vi "main_ai.vi"() -> ()   [LabVIEW 2023]
uses:
  <vilib>/sound2/lvsound2.llb/Sound Output Set Volume (Single).vi
panel:
  in  "Reset":bool
  out "p2 score":i32
  out "p1 score":i32
  in  "Ball Speed":dbl(slide)=2.0 scale=0.0..5.0
  in  "Player Length":i32(slide)=100 scale=50.0..150.0
  in  "Pause Game":bool
  in  "Stop":bool
  in  "w_bool":bool
  in  "Down_bool":bool
  in  "s_bool":bool
  in  "Up_bool":bool
  out "game window":picture
  # "Player 1: W, S\nPlayer 2: Up, Down"
  # "Modifiers"
  # "Spacebar"
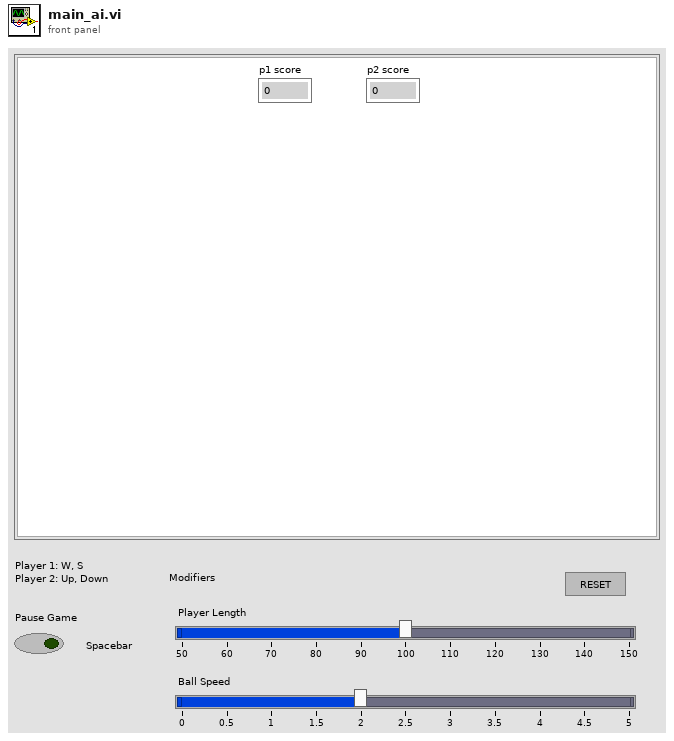
[diagram p1: front panel]
types:
  T1 = typedef "Sound Output Task ID.ctl" = u32
  T2 = cluster{"output vector x":dbl, "output vector y":dbl}
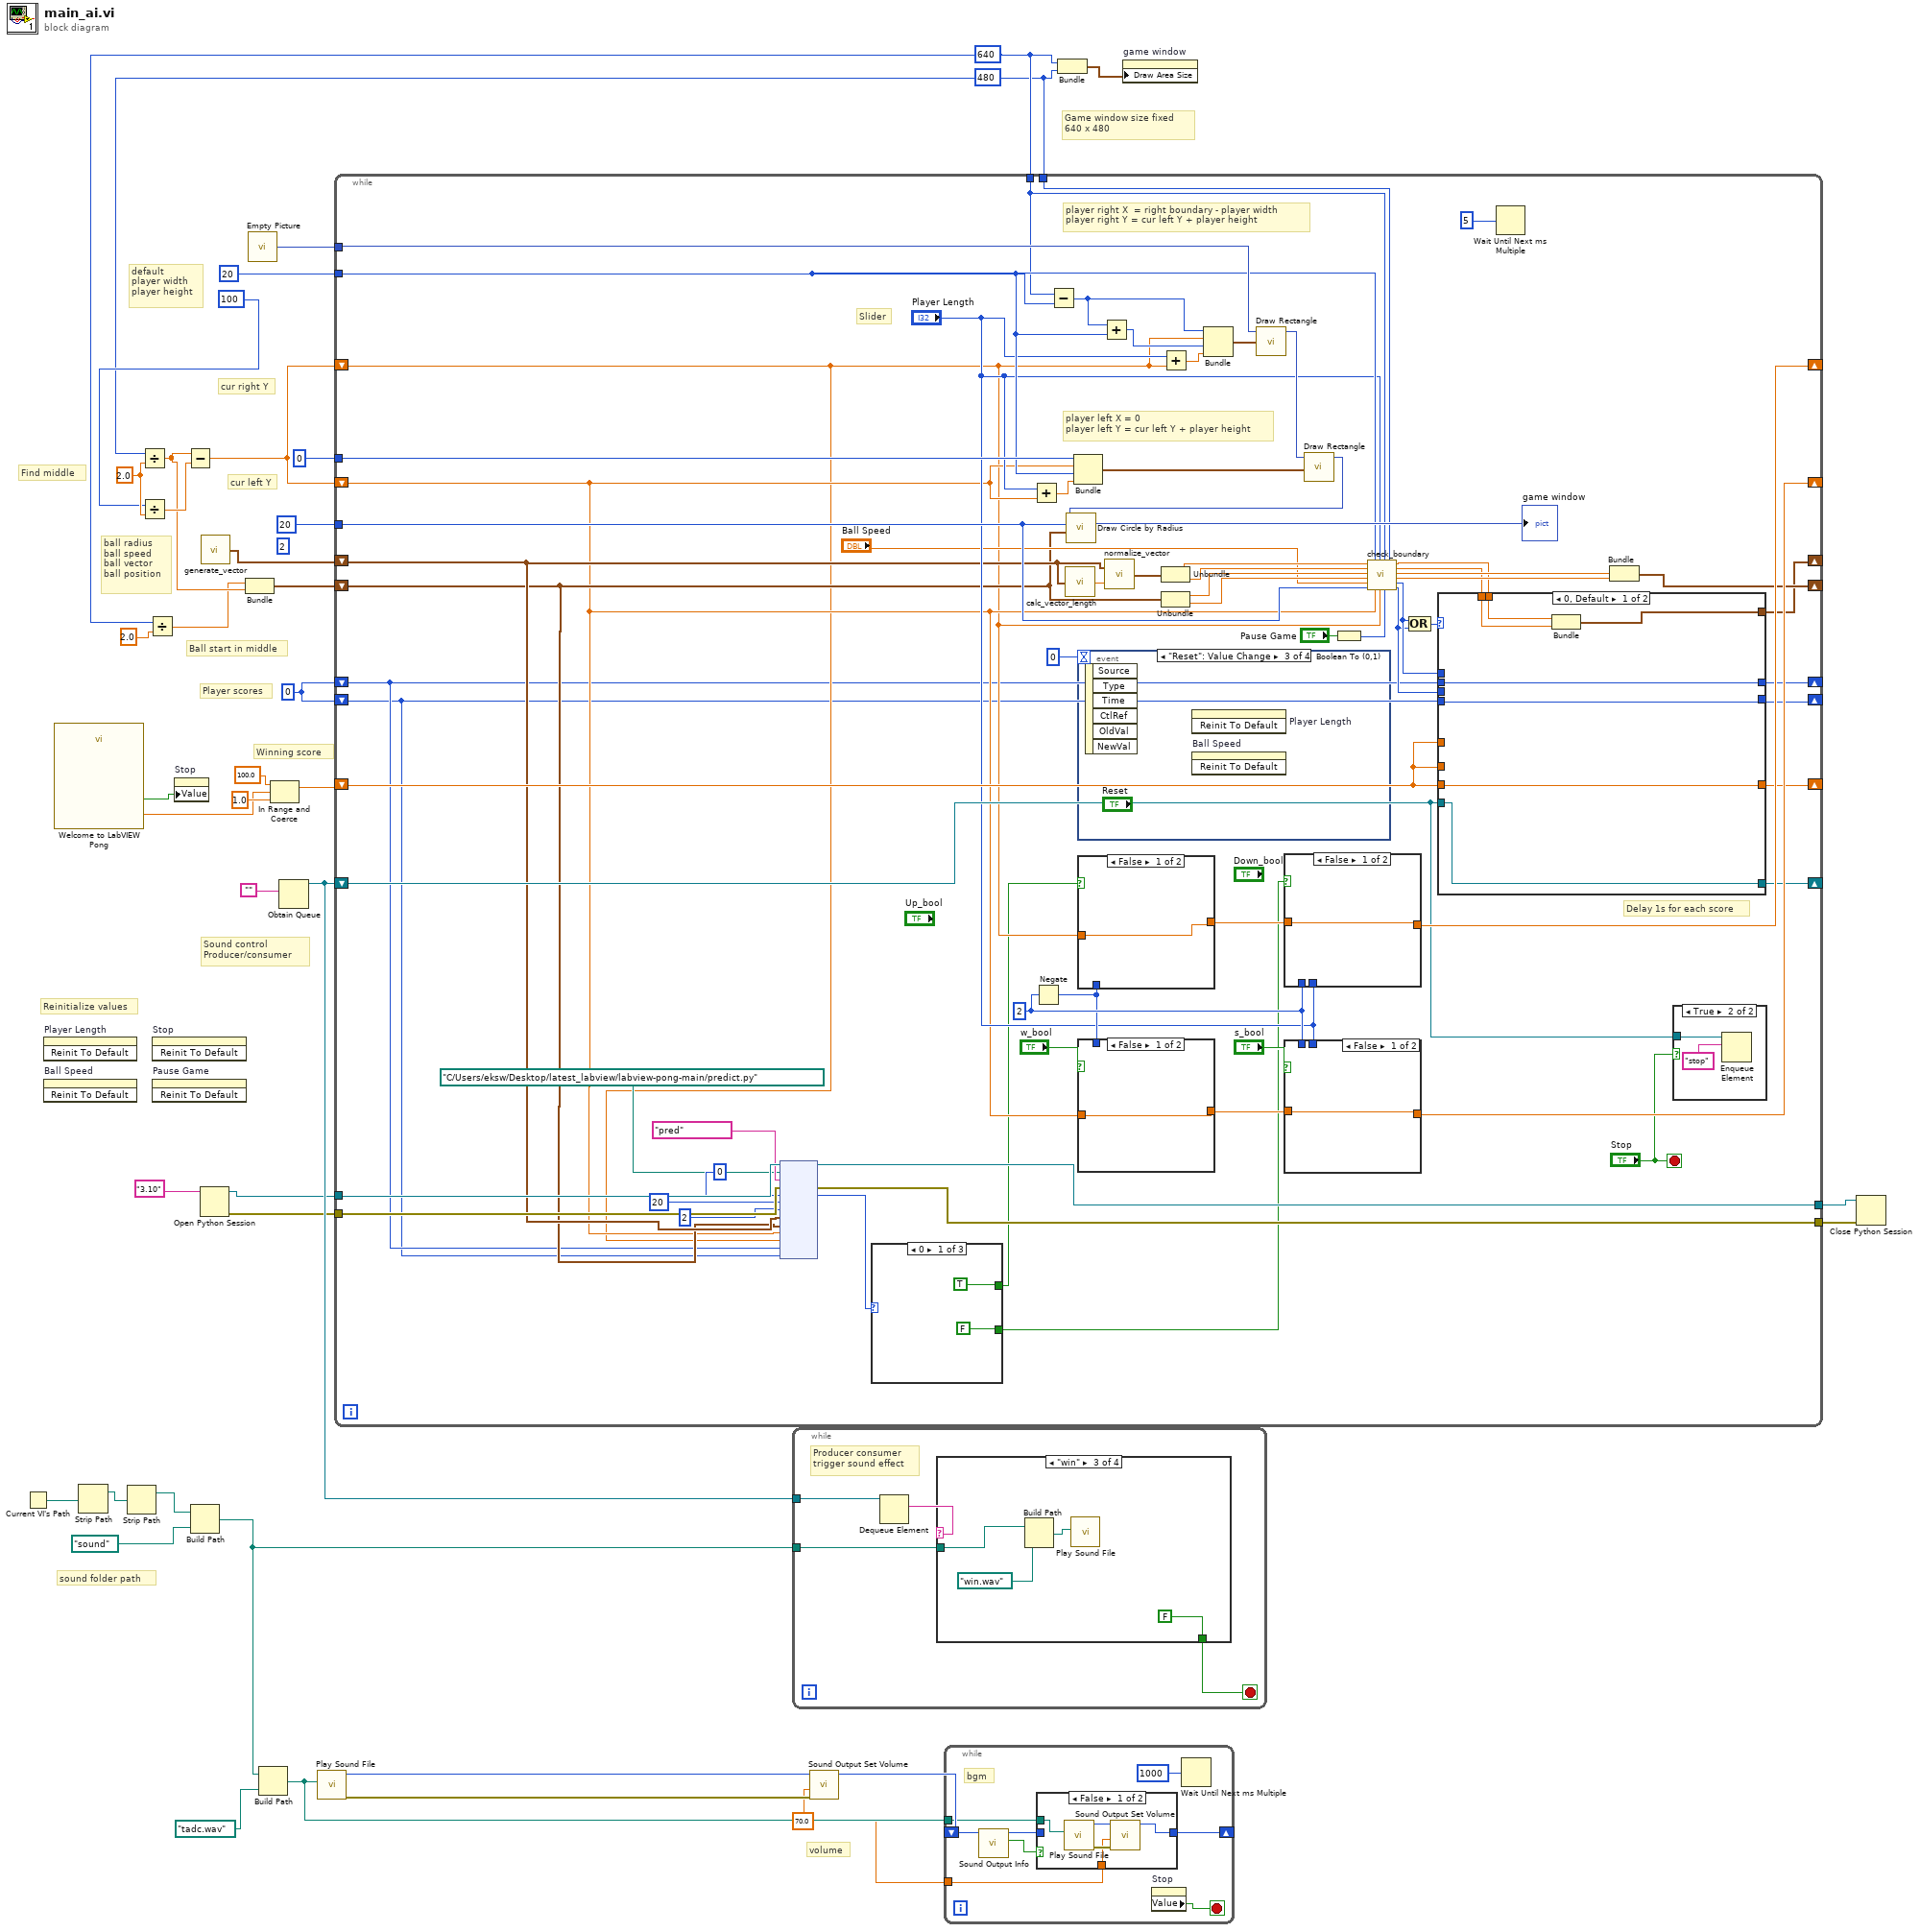
[diagram p0: block diagram]
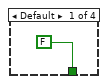
[diagram p3: hidden frame]
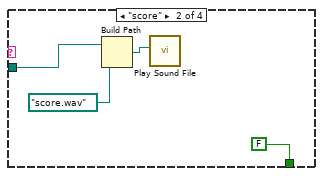
[diagram p4: hidden frame]
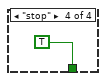
[diagram p5: hidden frame]
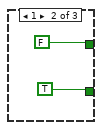
[diagram p6: hidden frame]
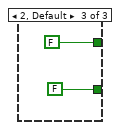
[diagram p7: hidden frame]
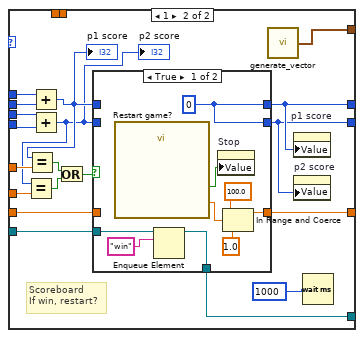
[diagram p9: hidden frame]
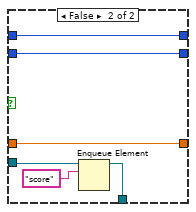
[diagram p10: hidden frame]
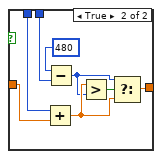
[diagram p11: hidden frame]
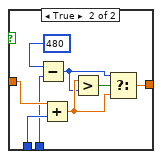
[diagram p12: hidden frame]
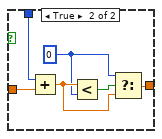
[diagram p13: hidden frame]
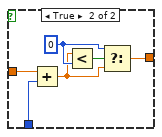
[diagram p14: hidden frame]
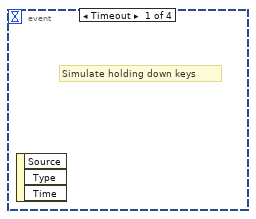
[diagram p15: hidden frame]
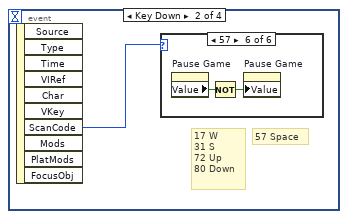
[diagram p16: hidden frame]
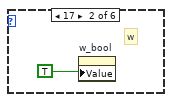
[diagram p18: hidden frame]
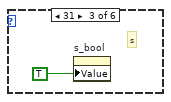
[diagram p19: hidden frame]
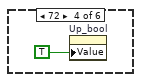
[diagram p20: hidden frame]
diagram:
  w7 = 70.0 ("volume")
  w25 = 0
  (unwired) 2
  w26 = 480
  w32 = 640
  w35 = 2.0 ("y")
  # "Reinitialize values"
  # "volume"
  # "sound folder path"
  # "Sound control\nProducer/consumer"
  # "Winning score"
  # "Player scores"
  # "Ball start in middle"
  # "ball radius\nball speed\nball vector\nball position"
  # "Find middle"
  # "default\nplayer width\nplayer height"
  # "cur left Y"
  # "cur right Y"
  # "Game window size fixed\n640 x 480"
  n1 = Current VI's Path() -> (path=w16:path)
  n2 = invoke on="Player Length" class="Slide (strict)" method="Reinit To Default"() -> ()  [unwired: 3 in, 3 out]
  n3 = invoke on="Ball Speed" class="Slide (strict)" method="Reinit To Default"() -> ()  [unwired: 3 in, 3 out]
  n4 = call "Welcome to LabVIEW Pong"() -> ("Winning Score"=w21:dbl, "Quit Game"=w6:bool)  [unwired: 17 in, 1 out]
  n5 = Strip Path(path=w16) -> (stripped path=w15:path)  [unwired: 1 out]
  n6 = Strip Path(path=w15) -> (stripped path=w17:path)  [unwired: 1 out]
  n7 = Divide(x=w26, y=w35) -> (x/y=w29:dbl)
  n8 = Divide(x=100, y=w35) -> (x/y=w34:dbl)
  n9 = Divide(x=w32, y=2.0) -> (x/y=w28:dbl)
  n10 = invoke on="Stop" class="Bool (strict)" method="Reinit To Default"() -> ()  [unwired: 3 in, 3 out]
  n11 = invoke on="Pause Game" class="Bool (strict)" method="Reinit To Default"() -> ()  [unwired: 3 in, 3 out]
  n12 = property on="Stop" class="Bool (strict)"("Value"=w6) -> ()  [unwired: 2 in, 2 out]
  n13 = Subtract(x=w29, y=w34) -> (x-y=w36:dbl)
  n14 = Build Path(base path=w17, name or relative path=path "sound") -> (appended path=w13:path)
  n15 = Open Python Session(python version="3.10" ("Python version")) -> (session out=w5:refnum<k35>, error out=w3:errorcluster)  [unwired: 2 in]
  n16 = call "generate_vector.vi"() -> ("Cluster"=w24:cluster{"number":dbl, "number":dbl})
  n17 = Bundle(w28, w29) -> (w30:cluster{dbl, dbl})  [unwired: 1 in]
  n18 = call "Empty Picture"() -> ("empty picture"=w39:picture)
  n19 = Build Path(base path=w13, name or relative path=path "tadc.wav") -> (appended path=w11:path)
  n20 = In Range and Coerce(upper limit=100.0, x=w21, lower limit=1.0) -> (coerced(x)=w22:dbl)  [unwired: 1 out]
  n21 = Obtain Queue(element data type="") -> (queue out=w12:refnum<queue>)  [unwired: 4 in, 2 out]
  n22 = call <vilib>:"Play Sound File.vi"("path"=w11) -> ("error out"=w9:errorcluster, "task ID"=w10:T1)  [unwired: 9 in]
  n23 = while {
    tunnel: w32 -> [w81]
    tunnel: w39 -> [w106]
    shift-right: [w95] -> _
    shift-left: w36 -> [w46]
    shift-right: [w93] -> _
    shift-left: w36 -> [w47]
    tunnel: 20 -> [w82]
    tunnel: 0 -> [w104]
    shift-right: [w70] -> _
    shift-left: w24 -> [w49]
    shift-right: [w77] -> _
    shift-left: w30 -> [w48]
    tunnel: 20 -> [w76]
    tunnel: w26 -> [w80]
    shift-right: [w75] -> _
    shift-left: w25 -> [w45]
    shift-right: [w74] -> _
    shift-left: w25 -> [w44]
    shift-right: [w73] -> _
    shift-left: w22 -> [w69]
    shift-right: [w63] -> _
    shift-left: w12 -> [w61]
    tunnel: w5 -> [w58]
    tunnel: [w57] -> w4
    tunnel: w3 -> [w56]
    tunnel: [w55] -> w2
    stop <- "Stop" stop-if-true
    w98 = 2 ("y")
    # "Slider"
    # "Delay 1s for each score"
    # "player right X  = right boundary - player width\nplayer right Y = cur left Y + player height"
    # "player left X = 0\nplayer left Y = cur left Y + player height"
    n24 = node(w58, path "C:/Users/eksw/Desktop/latest_labview/labview-pong-main/predict.py" ("module path"), "pred" ("function name"), w56, 0, 20, 2, w49, w48, w47, w46, w45, w44) -> (w57:refnum<k35>, w55:errorcluster, w43:i32)  [unwired: 8 in, 2 out]
    n25 = case shown="0" w43 {
      tunnel: [TRUE FALSE FALSE] -> w42
      tunnel: [FALSE TRUE FALSE] -> w41
      frame 0 {
      }
      frame 1 {
      }
      frame 2, Default {
      }
    }
    n26 = Add(x="Player Length", y=w47) -> (x+y=w103:dbl)
    n27 = Negate(x=w98) -> (-x=w97:i32)
    n28 = Subtract(x=w81, y=w82) -> (x-y=w109:i32)
    n29 = call "calc_vector_length.vi"("vector"=w49) -> ("length"=w87:dbl)
    n30 = Bundle(w104, w47, w82, w103) -> (w102:cluster{i32, dbl, i32, dbl})  [unwired: 1 in]
    n31 = event shown="[2] \"Reset\": Value Change" {
      selector: _ -> [_ _ _ _]
      dyn-events: _ -> [_ _ _ _]
      timeout: 0 -> [_ _ _ _]
      event Timeout {
        # "Simulate holding down keys"
        n32 = event-data() -> ()  [unwired: 1 in, 3 out]
      }
      event Key Down {
        # "57 Space"
        # "17 W\n31 S\n72 Up\n80 Down"
        n33 = event-data() -> ("ScanCode"=w191:i16)  [unwired: 1 in, 9 out]
        n34 = case shown="57" w191 {
          frame 0, Default {
          }
          frame 17 {
            # "w"
            n35 = property on="w_bool" class="Bool (strict)"("Value"=TRUE) -> ()  [unwired: 2 in, 2 out]
          }
          frame 31 {
            # "s"
            n36 = property on="s_bool" class="Bool (strict)"("Value"=TRUE) -> ()  [unwired: 2 in, 2 out]
          }
          frame 72 {
            n37 = property on="Up_bool" class="Bool (strict)"("Value"=TRUE) -> ()  [unwired: 2 in, 2 out]
          }
          frame 80 {
            n38 = property on="Down_bool" class="Bool (strict)"("Value"=TRUE) -> ()  [unwired: 2 in, 2 out]
          }
          frame 57 {
            n39 = property on="Pause Game" class="Bool (strict)"() -> ("Value"=w196:bool)  [unwired: 2 in, 2 out]
            n40 = Not(x=w196) -> (.not. x?=w197:bool)
            n41 = property on="Pause Game" class="Bool (strict)"("Value"=w197) -> ()  [unwired: 2 in, 2 out]
          }
        }
      }
      event "Reset": Value Change {
        n42 = event-data() -> ()  [unwired: 1 in, 6 out]
        n43 = invoke on="Player Length" class="Slide (strict)" method="Reinit To Default"() -> ()  [unwired: 3 in, 3 out]
        n44 = invoke on="Ball Speed" class="Slide (strict)" method="Reinit To Default"() -> ()  [unwired: 3 in, 3 out]
      }
      event Key Up {
        n45 = event-data() -> ("ScanCode"=w198:i16)  [unwired: 1 in, 5 out]
        n46 = case shown="72" w198 {
          frame 0, Default {
          }
          frame 17 {
            # "w"
            n47 = property on="w_bool" class="Bool (strict)"("Value"=FALSE) -> ()  [unwired: 2 in, 2 out]
          }
          frame 31 {
            # "s"
            n48 = property on="s_bool" class="Bool (strict)"("Value"=FALSE) -> ()  [unwired: 2 in, 2 out]
          }
          frame 72 {
            n49 = property on="Up_bool" class="Bool (strict)"("Value"=FALSE) -> ()  [unwired: 2 in, 2 out]
          }
          frame 80 {
            n50 = property on="Down_bool" class="Bool (strict)"("Value"=FALSE) -> ()  [unwired: 2 in, 2 out]
          }
        }
      }
    }
    n51 = case shown="False" w42 {
      tunnel: w97 -> [_ w186]
      tunnel: w46 -> [w184 w187]
      tunnel: [w184 w185] -> w96
      frame False {
      }
      frame True {
        w189 = 0 ("y")
        n52 = Add(x=w187, y=w186) -> (x+y=w188:dbl)
        n53 = Less?(x=w188, y=w189) -> (x < y?=w190:bool)
        n54 = Select(t=w189, s=w190, f=w188) -> (s? t:f=w185:dbl)
      }
    }
    n55 = case shown="False" "w_bool" {
      tunnel: w47 -> [w177 w179]
      tunnel: w97 -> [_ w180]
      tunnel: [w177 w178] -> w94
      frame False {
      }
      frame True {
        w181 = 0 ("y")
        n56 = Add(x=w180, y=w179) -> (x+y=w183:dbl)
        n57 = Less?(x=w183, y=w181) -> (x < y?=w182:bool)
        n58 = Select(t=w181, s=w182, f=w183) -> (s? t:f=w178:dbl)
      }
    }
    n59 = Add(x=w109, y=w82) -> (x+y=w108:i32)
    n60 = call "normalize_vector.vi"("Numeric"=w87, "vector"=w49) -> ("output"=w88:cluster{"x":dbl, "y":dbl})
    n61 = Unbundle(w88) -> ("x"=w86:dbl, "y"=w85:dbl)
    n62 = Unbundle(w48) -> (w84:dbl, w83:dbl)
    n63 = Add(x="Player Length", y=w46) -> (x+y=w107:dbl)
    n64 = Bundle(w109, w46, w108, w107) -> (w105:cluster{i32, dbl, i32, dbl})  [unwired: 1 in]
    n65 = call <vilib>:"Draw Rectangle.vi"("picture"=w106, "rect"=w105) -> ("new picture"=w101:picture)  [unwired: 7 in]
    n66 = case shown="False" w41 {
      tunnel: w98 -> [_ w172]
      tunnel: w96 -> [w168 w171]
      tunnel: [w168 w170] -> w95
      tunnel: "Player Length" -> [_ w169]
      frame False {
      }
      frame True {
        n67 = Subtract(x=480 ("y"), y=w169) -> (x-y=w174:i32)
        n68 = Add(x=w171, y=w172) -> (x+y=w175:dbl)
        n69 = Greater?(x=w175, y=w174) -> (0:w176:bool)
        n70 = Select(t=w174, s=w176, f=w175) -> (s? t:f=w170:dbl)
      }
    }
    n71 = case shown="False" "s_bool" {
      tunnel: w98 -> [_ w162]
      tunnel: w94 -> [w159 w163]
      tunnel: [w159 w161] -> w93
      tunnel: "Player Length" -> [_ w160]
      frame False {
      }
      frame True {
        n72 = Add(x=w162, y=w163) -> (x+y=w166:dbl)
        n73 = Subtract(x=480 ("y"), y=w160) -> (x-y=w165:i32)
        n74 = Greater?(x=w166, y=w165) -> (0:w167:bool)
        n75 = Select(t=w165, s=w167, f=w166) -> (s? t:f=w161:dbl)
      }
    }
    n76 = call <vilib>:"Draw Rectangle.vi"("picture"=w101, "rect"=w102) -> ("new picture"=w90:picture)  [unwired: 7 in]
    n77 = call <vilib>:"Draw Circle by Radius.vi"("pixel center"=w48, "radius"=w76, "picture"=w90) -> ("new picture"=→"game window":picture)  [unwired: 8 in]
    n78 = Boolean To (0,1)(Boolean="Pause Game") -> (0, 1=w64:i16)
    n79 = call "check_boundary.vi"("vector x"=w86, "vector y"=w85, "position x"=w84, "position y"=w83, "speed"="Ball Speed", "radius"=w76, "player width"=w82, "player left position y"=w47, "player height"="Player Length", "player right position y"=w46, "window width"=w81, "pause"=w64, "window height"=w80) -> ("output vector x"=w72:dbl, "output vector y"=w71:dbl, "output x"=w79:dbl, "output y"=w78:dbl, "left win"=w67:i32, "right win"=w66:i32)  [unwired: 1 in]
    n80 = Compound Arithmetic op=OR(w67, w66) -> (w68:i32)
    n81 = case shown="0, Default" w68 {
      tunnel: w45 -> [w124 w134]
      tunnel: w44 -> [w123 w132]
      tunnel: w67 -> [_ w135]
      tunnel: w66 -> [_ w133]
      tunnel: [w124 w128] -> w75
      tunnel: [w123 w127] -> w74
      tunnel: w69 -> [_ w143]
      tunnel: w69 -> [_ w142]
      tunnel: [w122 w138] -> w73
      tunnel: w69 -> [w122 w137]
      tunnel: w72 -> [w121 _]
      tunnel: w71 -> [w120 _]
      tunnel: [w119 w136] -> w70
      tunnel: w61 -> [w118 w126]
      tunnel: [w118 w125] -> w63
      frame 0, Default {
        n82 = Bundle("output vector x"=w121, "output vector y"=w120) -> (w119:T2)  [unwired: 1 in]
      }
      frame 1 {
        # "Scoreboard\nIf win, restart?"
        n83 = Add(x=w135, y=w134) -> (x+y=w130:i32)
        "p1 score" <- w130
        n84 = Equal?(x=w130, y=w143) -> (x = y?=w140:bool)
        n85 = Add(x=w133, y=w132) -> (x+y=w129:i32)
        "p2 score" <- w129
        n86 = Equal?(x=w129, y=w142) -> (x = y?=w139:bool)
        n87 = Or(x=w140, y=w139) -> (x .or. y?=w141:bool)
        n88 = case shown="True" w141 {
          tunnel: [w151 w156] -> w127
          tunnel: [w151 w157] -> w128
          tunnel: [w148 w158] -> w138
          tunnel: w137 -> [_ w158]
          tunnel: w130 -> [_ w157]
          tunnel: w129 -> [_ w156]
          tunnel: w126 -> [w146 w154]
          tunnel: [w144 w153] -> w125
          frame True {
            w151 = 0
            n89 = call "Restart game?"() -> ("Winning Score"=w147:dbl, "Quit game"=w152:bool)  [unwired: 17 in, 1 out]
            n90 = Enqueue Element(queue=w146, element="win") -> (queue out=w144:refnum<queue>)  [unwired: 2 in, 2 out]
            n91 = property on="Stop" class="Bool (strict)"("Value"=w152) -> ()  [unwired: 2 in, 2 out]
            n92 = In Range and Coerce(upper limit=100.0, x=w147, lower limit=1.0) -> (coerced(x)=w148:dbl)  [unwired: 1 out]
          }
          frame False {
            n93 = Enqueue Element(queue=w154, element="score") -> (queue out=w153:refnum<queue>)  [unwired: 2 in, 2 out]
          }
        }
        n94 = call "generate_vector.vi"() -> ("Cluster"=w136:cluster{"number":dbl, "number":dbl})
        n95 = property on="p1 score" class="DigNum (strict)"("Value"=w128) -> ()  [unwired: 2 in, 2 out]
        n96 = property on="p2 score" class="DigNum (strict)"("Value"=w127) -> ()  [unwired: 2 in, 2 out]
        n97 = Wait (ms)(milliseconds to wait=u32 1000) -> ()  [unwired: 1 out]
      }
    }
    n98 = Wait Until Next ms Multiple(millisecond multiple=u32 5 ("milliseconds to wait")) -> ()  [unwired: 1 out]
    n99 = Bundle("output x"=w79, "output y"=w78) -> (w77:cluster{"output x":dbl, "output y":dbl})  [unwired: 1 in]
    n100 = case shown="True" "Stop" {
      tunnel: w61 -> [_ w117]
      frame False {
      }
      frame True {
        n101 = Enqueue Element(queue=w117, element="stop") -> ()  [unwired: 2 in, 3 out]
      }
    }
  }
  n102 = while {
    tunnel: w12 -> [w206]
    tunnel: w13 -> [w204]
    stop <- w203 stop-if-true
    # "Producer consumer\ntrigger sound effect"
    n103 = Dequeue Element(queue=w206) -> (element=w205:string)  [unwired: 2 in, 3 out]
    n104 = case shown="\"win\"" w205 {
      tunnel: w204 -> [_ w211 w215 _]
      tunnel: [FALSE ("Stop") FALSE ("Stop") FALSE ("Stop") TRUE ("Stop")] -> w203
      frame Default {
      }
      frame "score" {
        n105 = Build Path(base path=w211, name or relative path=path "score.wav") -> (appended path=w208:path)
        n106 = call <vilib>:"Play Sound File.vi"("path"=w208) -> ()  [unwired: 9 in, 2 out]
      }
      frame "win" {
        n107 = Build Path(base path=w215, name or relative path=path "win.wav") -> (appended path=w212:path)
        n108 = call <vilib>:"Play Sound File.vi"("path"=w212) -> ()  [unwired: 9 in, 2 out]
      }
      frame "stop" {
      }
    }
  }
  n109 = call-poly <vilib>:"Sound Output Set Volume.vi"("error in (no error)"=w9, "volume"=w7, "task ID"=w10) -> ("task ID out"=w8:T1)  [unwired: 7 in, 1 out]
  n110 = while {
    shift-right: [w220] -> _
    shift-left: w8 -> [w222]
    tunnel: w11 -> [w218]
    tunnel: w7 -> [w217]
    stop <- w223 stop-if-true
    # "bgm"
    n111 = call <vilib>:"Sound Output Info.vi"("task ID"=w222) -> ("is playing?"=w221:bool, "task ID out"=w219:T1)  [unwired: 7 in, 2 out]
    n112 = case shown="False" w221 {
      tunnel: [w226 w230] -> w220
      tunnel: w219 -> [_ w230]
      tunnel: w218 -> [w229 _]
      tunnel: w217 -> [w225 _]
      frame False {
        n113 = call <vilib>:"Play Sound File.vi"("path"=w229) -> ("error out"=w228:errorcluster, "task ID"=w227:T1)  [unwired: 9 in]
        n114 = call-poly <vilib>:"Sound Output Set Volume.vi"("error in (no error)"=w228, "volume"=w225, "task ID"=w227) -> ("task ID out"=w226:T1)  [unwired: 7 in, 1 out]
      }
      frame True {
      }
    }
    n115 = property on="Stop" class="Bool (strict)"() -> ("Value"=w223:bool)  [unwired: 2 in, 2 out]
    n116 = Wait Until Next ms Multiple(millisecond multiple=u32 1000) -> ()  [unwired: 1 out]
  }
  n117 = Bundle(w32, w26) -> (w40:cluster{i32, i32})  [unwired: 1 in]
  n118 = property on="game window" class="Pict"("Draw Area Size"=w40) -> ()  [unwired: 2 in, 2 out]
  n119 = Close Python Session(session in=w4, error in=w2) -> ()  [unwired: 1 out]
